vi "Laser-Set-Parmeter-new.vi"(2 "error in (no error)":errorcluster, 3 "LaserHV":u8=20, 5 "LaserFreq":u8=60, 6 "SetTransmission":i16=1 min=0 max=100, 7 "VISA resource name":refnum<visa-resource-name>) -> (0 "error out":errorcluster, 1 "VISA resource name out":refnum<visa-resource-name>)   [LabVIEW 2013]
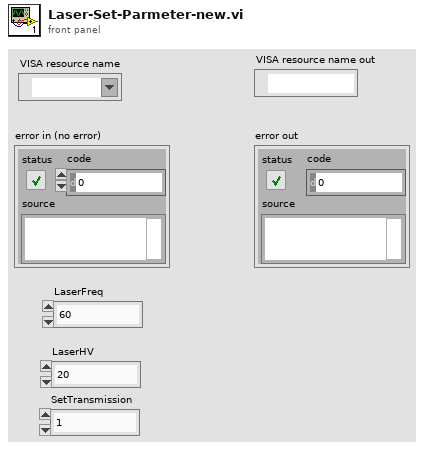
[diagram p1: front panel]
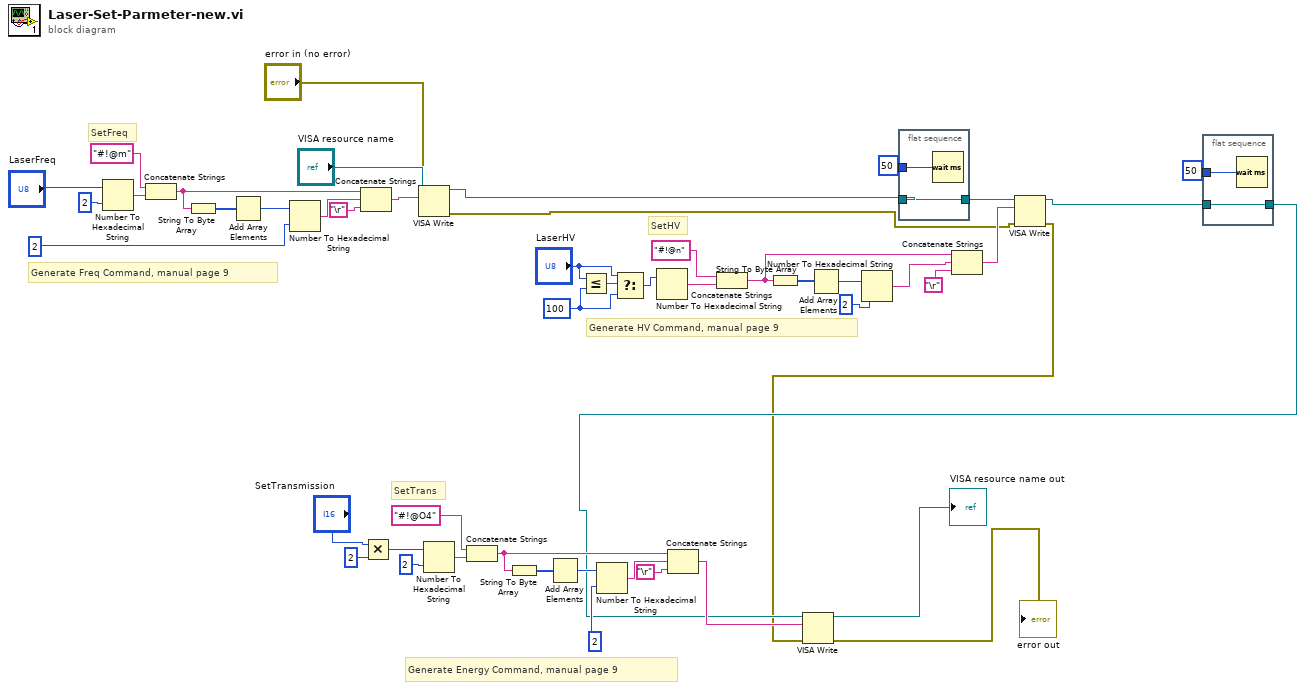
[diagram p0: block diagram]
diagram:
  w36 = u8 100 ("y")
  # "Generate Energy Command, manual page 9"
  # "SetTrans"
  # "Generate HV Command, manual page 9"
  # "Generate Freq Command, manual page 9"
  # "SetHV"
  # "SetFreq"
  n1 = Number To Hexadecimal String(1:i16 2 ("width (-)"), 2:"LaserFreq") -> (0:w46:string)
  n2 = Concatenate Strings("#!@m" ("string"), w46) -> (w42:string)
  n3 = String To Byte Array(string=w42) -> (unsigned byte array=w45:u8[])
  n4 = Add Array Elements(numeric array=w45) -> (sum=w44:u8)
  n5 = Number To Hexadecimal String(1:i16 2 ("width (-)"), 2:w44) -> (0:w41:string)
  n6 = Concatenate Strings(w42, w41, "\r") -> (w39:string)
  n7 = Multiply(x="SetTransmission", y=2) -> (x*y=w17:i32)
  n8 = VISA Write(VISA resource name="VISA resource name", write buffer=w39, error in (no error)="error in (no error)") -> (VISA resource name out=w25:refnum<visa-resource-name>, error out=w18:errorcluster)  [unwired: 1 out]
  n9 = Number To Hexadecimal String(1:i16 2 ("width (-)"), 2:w17) -> (0:w9:string)
  n10 = Concatenate Strings("#!@O4" ("string"), w9) -> (w13:string)
  n11 = String To Byte Array(string=w13) -> (unsigned byte array=w10:u8[])
  n12 = Add Array Elements(numeric array=w10) -> (sum=w11:u8)
  n13 = Less Or Equal?(x="LaserHV", y=w36) -> (x <= y?=w38:bool)
  n14 = Number To Hexadecimal String(1:i16 2 ("width (-)"), 2:w11) -> (0:w14:string)
  n15 = Select(t="LaserHV", s=w38, f=w36) -> (s? t:f=w27:u8)
  n16 = Number To Hexadecimal String(2:w27) -> (0:w34:string)  [unwired: 1 in]
  n17 = Concatenate Strings(w13, w14, "\r") -> (w5:string)
  n18 = Concatenate Strings("#!@n" ("string"), w34) -> (w30:string)
  n19 = String To Byte Array(string=w30) -> (unsigned byte array=w33:u8[])
  n20 = Add Array Elements(numeric array=w33) -> (sum=w32:u8)
  n21 = Number To Hexadecimal String(1:i16 2 ("width (-)"), 2:w32) -> (0:w29:string)
  n22 = flat-sequence {
    tunnel: w25 -> [w50]
    tunnel: [w50] -> w24
    tunnel: u32 50 ("delay before read (ms)") -> [w51]
    frame #0 {
      n23 = Wait (ms)(milliseconds to wait=w51) -> ()  [unwired: 1 out]
    }
  }
  n24 = Concatenate Strings(w30, w29, "\r") -> (w23:string)
  n25 = VISA Write(VISA resource name=w24, write buffer=w23, error in (no error)=w18) -> (VISA resource name out=w21:refnum<visa-resource-name>, error out=w2:errorcluster)  [unwired: 1 out]
  n26 = VISA Write(VISA resource name=w4, write buffer=w5, error in (no error)=w2) -> (VISA resource name out=→"VISA resource name out":refnum<visa-resource-name>, error out=→"error out":errorcluster)  [unwired: 1 out]
  n27 = flat-sequence {
    tunnel: w21 -> [w52]
    tunnel: [w52] -> w4
    tunnel: u32 50 ("delay before read (ms)") -> [w53]
    frame #0 {
      n28 = Wait (ms)(milliseconds to wait=w53) -> ()  [unwired: 1 out]
    }
  }
